vi "Get Next.vi"(0 "Subsequence in":refnum<class "Subsequence.lvclass">, 1 "Linked List Ref":refnum<data-value>, 5 "Active Unique ID":string, 9 "Active Element Index":i32, 11 "error in (no error)":errorcluster) -> (3 "Linked List Ref out":refnum<data-value>, 4 "Executioner out":refnum<class "Executioner.lvclass">, 6 "Active Unique ID out":string, 8 "Test Executive Ref out":refnum<data-value>, 10 "Active Element Index out":i32, 12 "Found":bool, 13 "Complete":bool, 14 "Stop":bool, 15 "error out":errorcluster)   [LabVIEW 2019, in "Test Executive.lvlib" / "Subsequence.lvclass"]
uses:
  <vilib>/gpm_packages/@cs/test-executive/Source/Test Executive/Subsequence/Subsequence.lvclass
  C:/Program Files/National Instruments/LabVIEW 2019/vi.lib/gpm_packages/@cs/test-executive/Source/Test Executive/Executioner/Executioner.lvclass
  <vilib>/gpm_packages/@cs/test-executive/Source/Test Executive/Executioner/Executioner.lvclass
  <vilib>/gpm_packages/@cs/linked-list/Source/Linked List/ILinkedList/ILinked List.lvclass
  <vilib>/gpm_packages/@cs/test-executive/Source/Test Executive/ITestExecutive/ITest Executive.lvclass
  <vilib>/gpm_packages/@cs/linked-list/Source/Linked List/Linked List Ref/Linked List Ref.lvclass
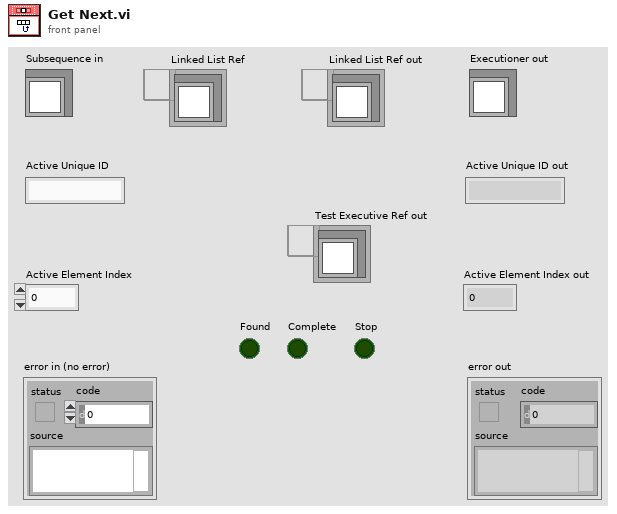
[diagram p1: front panel]
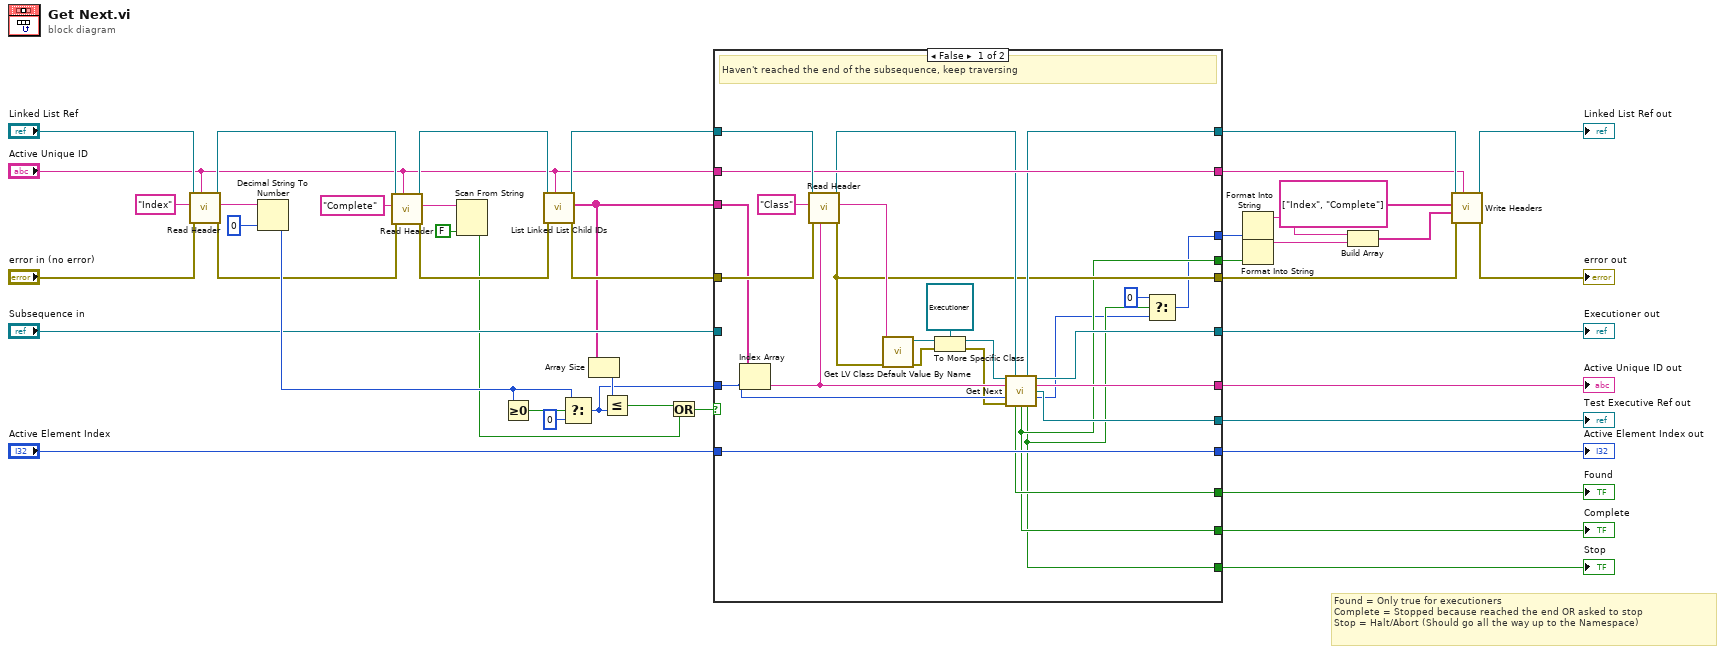
[diagram p0: block diagram]
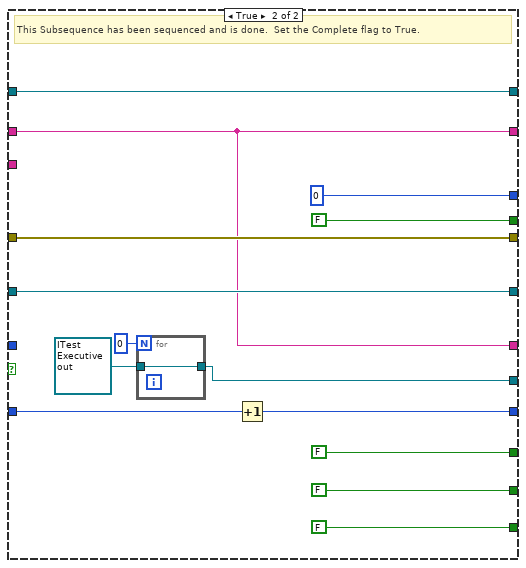
[diagram p2: hidden frame]
diagram:
  # "Found = Only true for executioners\nComplete = Stopped because reached the end OR asked to stop\nStop = Halt/Abort (Should go all the way up to the Namespace)"
  n1 = call <vilib>:"Read Header.vi"("Linked List ID"="Active Unique ID", "error in (no error)"="error in (no error)", "Header Name"="Index" ("Attribute Name"), "Linked List Ref"="Linked List Ref") -> ("error out"=w4:errorcluster, "Header Value"=w17:string, "Linked List Ref out"=w7:refnum<data-value>)  [unwired: 4 in, 1 out]
  n2 = Decimal String To Number(string=w17, default (0L)=0 ("Attribute")) -> (number=w39:i32)  [unwired: 1 in, 1 out]
  n3 = call <vilib>:"Read Header.vi"("Linked List ID"="Active Unique ID", "error in (no error)"=w4, "Header Name"="Complete" ("Attribute Name"), "Linked List Ref"=w7) -> ("error out"=w3:errorcluster, "Header Value"=w9:string, "Linked List Ref out"=w6:refnum<data-value>)  [unwired: 4 in, 1 out]
  n4 = Scan From String(input string=w9, default 1=FALSE) -> (output 1=w2:bool)  [unwired: 3 in, 3 out]
  n5 = Greater Or Equal To 0?(x=w39) -> (x >= 0?=w42:bool)
  n6 = call <vilib>:"List Linked List Child IDs.vi"("Linked List ID"="Active Unique ID", "error in (no error)"=w3, "Linked List Ref"=w6) -> ("error out"=w37:errorcluster, "Child IDs"=w20:string[], "Linked List Ref out"=w38:refnum<data-value>)  [unwired: 6 in]
  n7 = Select(t=w39, s=w42, f=0) -> (s? t:f=w36:i32)
  n8 = Array Size(array=w20) -> (size(s)=w40:i32)
  n9 = Less Or Equal?(x=w40, y=w36) -> (x <= y?=w19:bool)
  n10 = Or(x=w19, y=w2) -> (x .or. y?=w1:bool)
  n11 = case shown="False" w1 {
    tunnel: [w64 w84] -> w27
    tunnel: w38 -> [w70 w84]
    tunnel: [w56 w83] -> w26
    tunnel: w37 -> [w69 w83]
    tunnel: w36 -> [w63 _]
    tunnel: "Active Element Index" -> [w54 w81]
    tunnel: [w67 w76] -> w22
    tunnel: "Active Unique ID" -> [w67 w76]
    tunnel: [w51 w82] -> w34
    tunnel: "Subsequence in" -> [_ w82]
    tunnel: [w54 w80] -> w32
    tunnel: [w53 FALSE] -> w31
    tunnel: [w49 FALSE] -> w30
    tunnel: [w47 FALSE] -> w29
    tunnel: [w52 w76] -> w28
    tunnel: [w45 0] -> w25
    tunnel: [w49 FALSE] -> w21
    tunnel: w20 -> [w66 _]
    tunnel: [w50 w71] -> w11
    frame False {
      # "Haven't reached the end of the subsequence, keep traversing"
      n12 = Index Array(array=w66, index=w63) -> (element=w62:string)
      n13 = call <vilib>:"Read Header.vi"("Linked List ID"=w62, "error in (no error)"=w69, "Header Name"="Class", "Linked List Ref"=w70) -> ("error out"=w56:errorcluster, "Header Value"=w61:string, "Linked List Ref out"=w65:refnum<data-value>)  [unwired: 4 in, 1 out]
      n14 = call <vilib>:"Get LV Class Default Value By Name.vi"("error in (no error)"=w56, "class name"=w61) -> ("error out"=w57:errorcluster, "object"=w60:refnum<class>)  [unwired: 8 in]
      n15 = To More Specific Class(target class=refnum<class "Executioner.lvclass"> refnum ("Test Executive.lvlib:Executioner.lvclass"), reference=w60, error in=w57) -> (specific class reference=w55:refnum<class "Executioner.lvclass">, error out=w58:errorcluster)
      n16 = call-dynamic "Get Next.vi"("Executioner in"=w55, "Linked List Ref"=w65, "Active Unique ID"=w62, "Active Element Index"=w63, "error in (no error)"=w58) -> ("Linked List Ref out"=w64:refnum<data-value>, "Executioner out"=w51:refnum<class "Executioner.lvclass">, "Active Unique ID out"=w52:string, "Test Executive Ref out"=w50:refnum<data-value>, "Active Element Index out"=w46:i32, "Found"=w53:bool, "Complete"=w49:bool, "Stop"=w47:bool)  [unwired: 2 in, 1 out]
      n17 = Select(t=0, s=w47, f=w46) -> (s? t:f=w45:i32)
    }
    frame True {
      # "This Subsequence has been sequenced and is done.  Set the Complete flag to True."
      n18 = for {
        N: 0 -> [_]
        tunnel: refnum<data-value> refnum ("Test Executive Ref out") -> [w85]
        tunnel: [w85] -> w71
      }
      n19 = Increment(x=w81) -> (x+1=w80:i32)
    }
  }
  "Executioner out" <- w34
  "Active Unique ID out" <- w28
  "Active Element Index out" <- w32
  "Found" <- w31
  "Complete" <- w30
  "Stop" <- w29
  "Test Executive Ref out" <- w11
  n20 = Format Into String(w25) -> (resulting string=w14:string)  [unwired: 3 in, 1 out]
  n21 = Format Into String(w21) -> (resulting string=w13:string)  [unwired: 3 in, 1 out]
  n22 = Build Array(w14, w13) -> (w12:string[])
  n23 = call <vilib>:"Write Headers.vi"("Linked List ID"=w22, "error in (no error)"=w26, "Header Values"=w12, "Header Names"=string[] ["Index", "Complete"], "Linked List Ref"=w27) -> ("error out"=→"error out":errorcluster, "Linked List Ref out"=→"Linked List Ref out":refnum<data-value>)  [unwired: 5 in]
